vi "Pagina gestione password.vi"() -> (0 "pagina out":i16=255)   [LabVIEW 2022 SP3]
uses:
  Labview/Globali.vi
  <vilib>/Utility/file.llb/Read From Spreadsheet File (string).vi
  <vilib>/Utility/file.llb/Write To Spreadsheet File (string).vi
panel:
  in  "Informazioni operatore 2":T1
  out "Manutenzione":string
  out "Autocontrollo Man.":string
  out "Password Man.":string
  out "Password Amm.":string
  out "Autocontrollo Amm.":string
  out "Amministratore":string
  in  "Informazioni operatore":T1
  in  "Aggiungi":bool
  in  "Informazioni operatori":T2(array[cluster])
  in  "stop":bool
  out "Password":string
  out "Autocontrollo":string
  out "Operatore":string
  out "Tipo pagina":string
  out "Indicazioni":string
  out "Picture":picture
  out "Versione SW":dbl=1.0 format="%.2f"
  out "Linea":string="CENTAURO"
  out "Testo allarmi":string caption="ALLARMI"
  out "Testo fase collaudo":string caption="FASE COLLAUDO"
  out "Testo segnalazioni":string caption="SEGNALAZIONI"
  out "Testo messaggi":string caption="MESSAGGI"
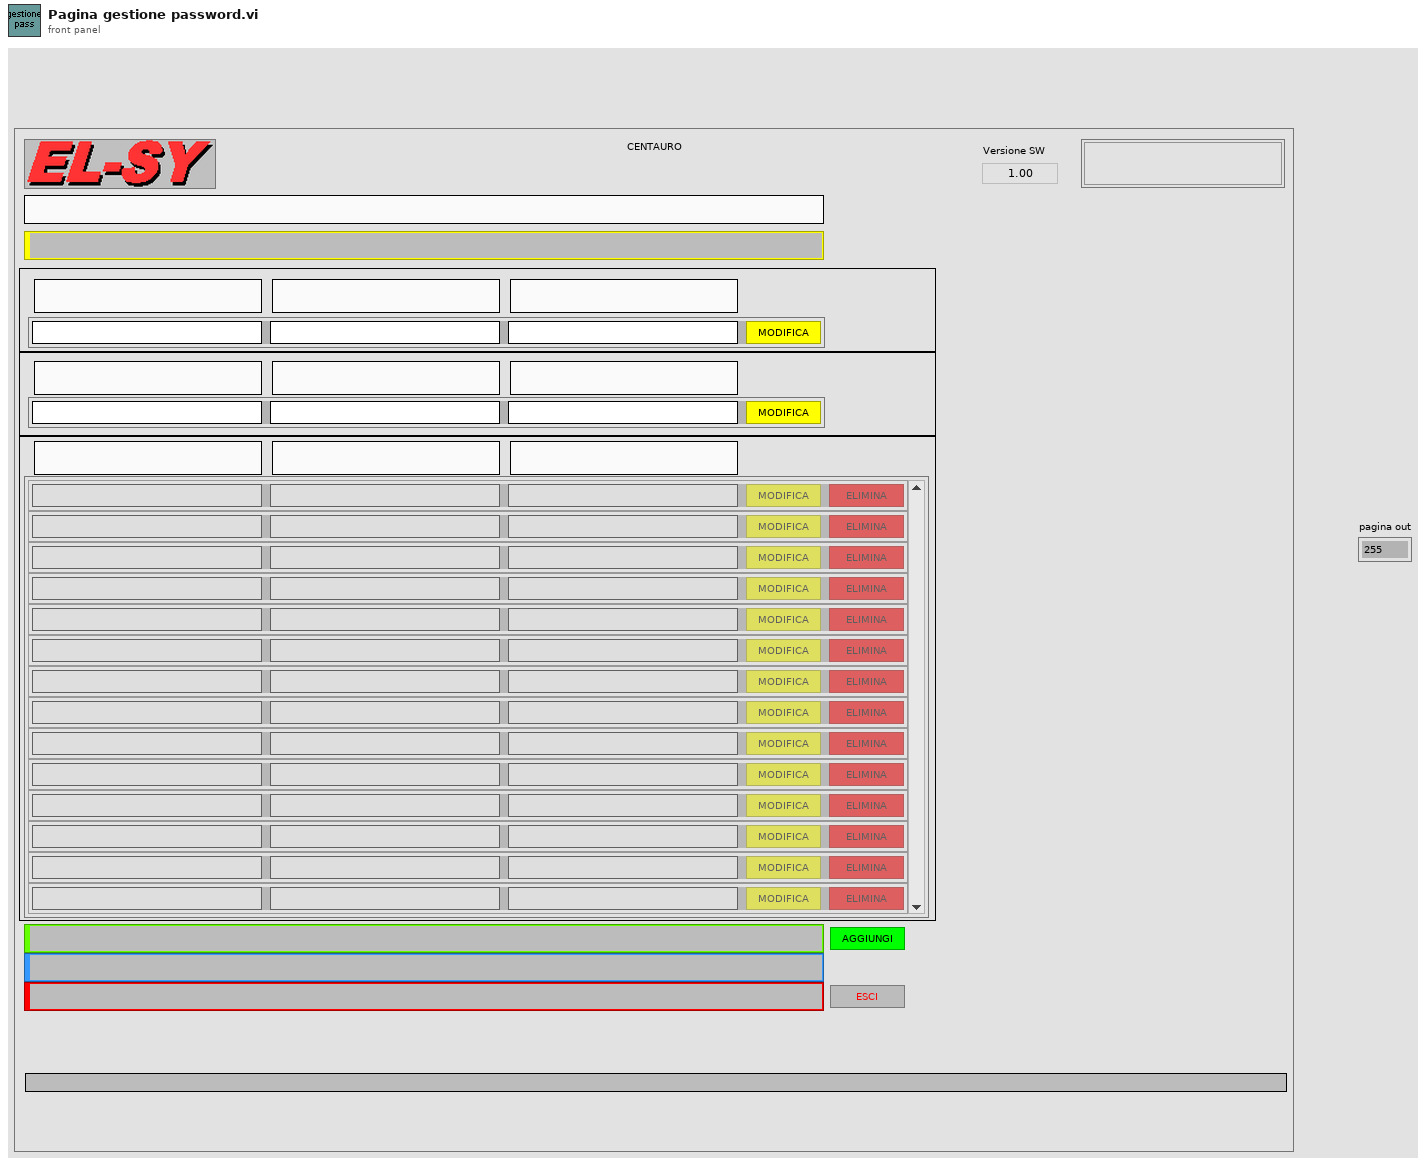
[diagram p1: front panel]
types:
  T1 = cluster{"Operatore":string, "Autocontrollo":string, "Password":string, "Aggiungi":bool, "Modifica":bool, "Elimina":bool}
  T2 = cluster{"Operatore":string, "Autocontrollo":string, "Password":string, "Aggiungi":bool, "Modifica":bool, "Elimina":bool}[]
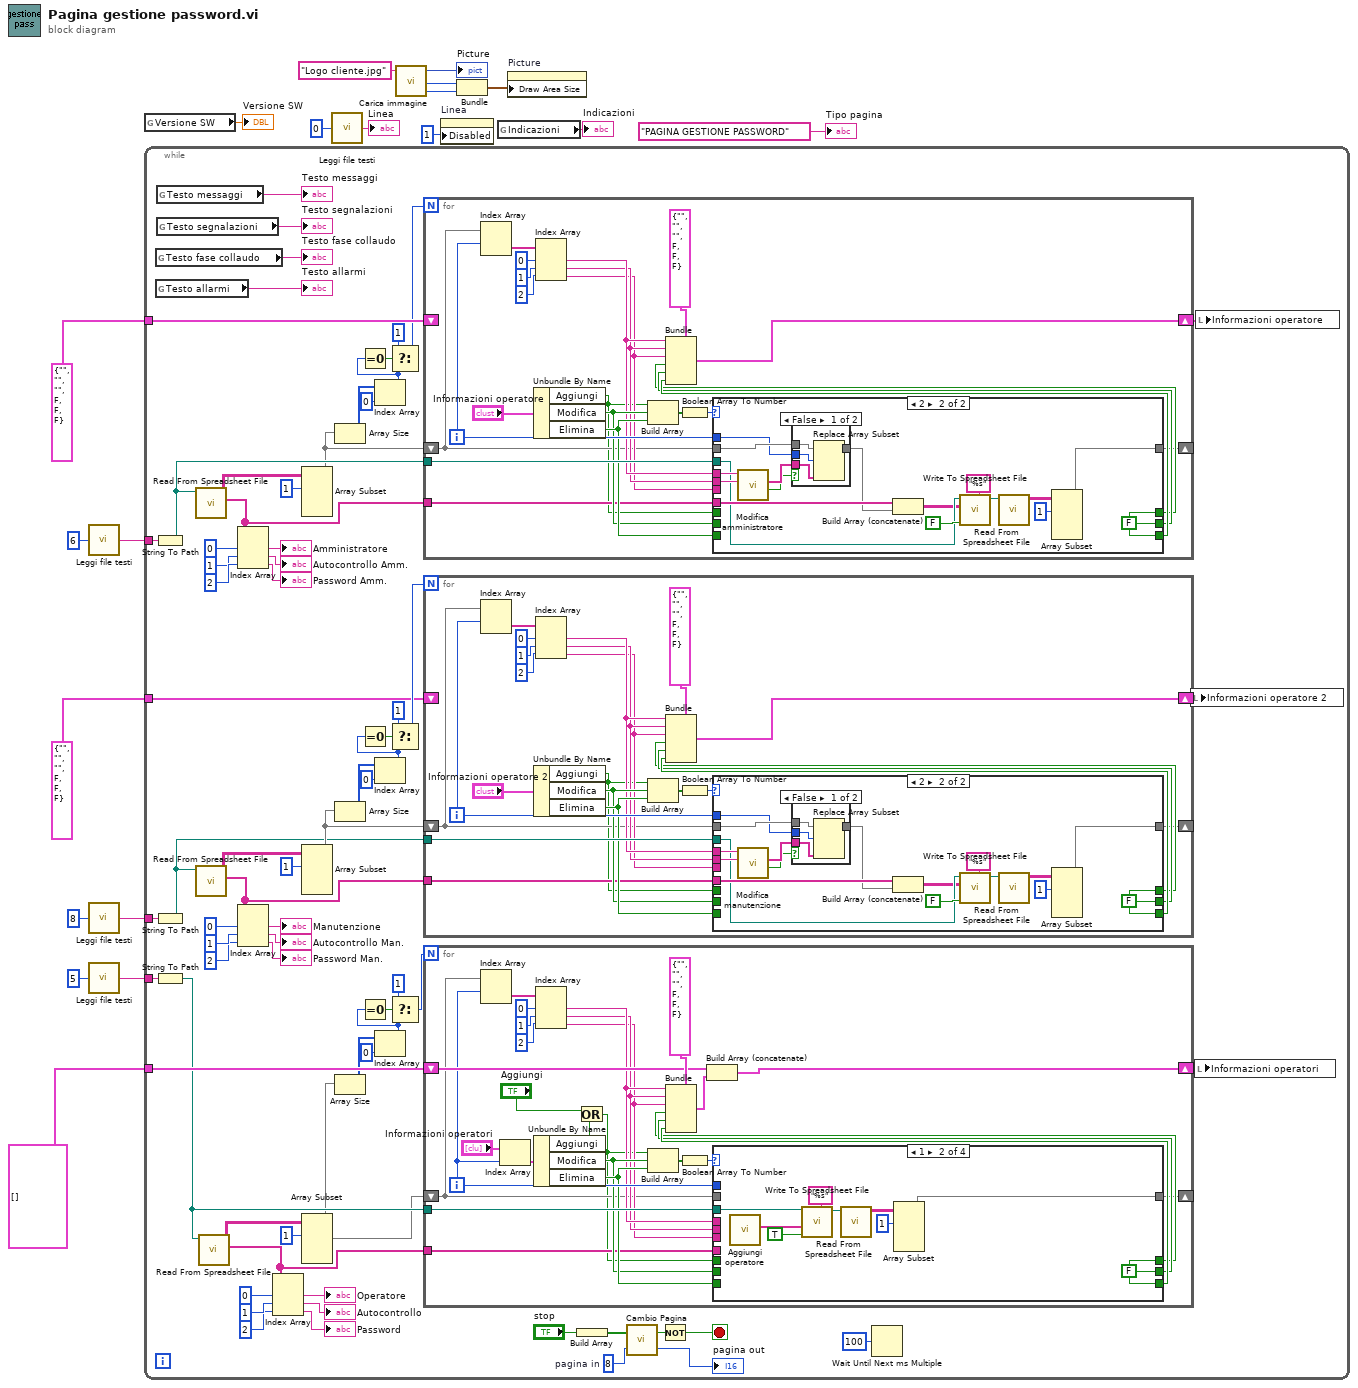
[diagram p0: block diagram]
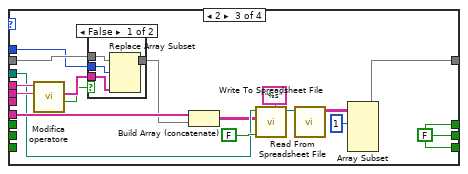
[diagram p7: hidden frame]
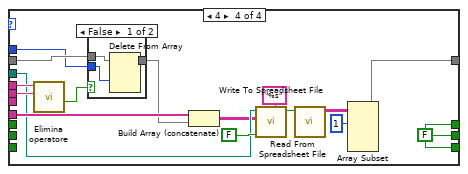
[diagram p9: hidden frame]
diagram:
  n1 = call "Leggi file testi.vi"("Numero riga"=6) -> ("Testo"=w7:string)  [unwired: 3 in, 1 out]
  n2 = call "Leggi file testi.vi"("Numero riga"=8) -> ("Testo"=w1:string)  [unwired: 3 in, 1 out]
  n3 = call "Leggi file testi.vi"("Numero riga"=5) -> ("Testo"=w8:string)  [unwired: 3 in, 1 out]
  n4 = global read "globali.vi" "Versione SW"() -> (→"Versione SW":dbl)
  n5 = while {
    tunnel: w8 -> [w83]
    tunnel: T2 [] ("Informazioni operatori 2") -> [w82]
    tunnel: w7 -> [w61]
    tunnel: T1 {"Operatore"="", "Autocontrollo"="", "Password"="", "Aggiungi"=FALSE, "Modifica"=FALSE, "Elimina"=FALSE} ("Informazioni operatore") -> [w49]
    tunnel: w1 -> [w21]
    tunnel: T1 {"Operatore"="", "Autocontrollo"="", "Password"="", "Aggiungi"=FALSE, "Modifica"=FALSE, "Elimina"=FALSE} ("Informazioni operatore") -> [w32]
    stop <- w62 stop-if-true
    w88 = u8 8  # pagina in
    n6 = String To Path(string=w61) -> (path=w55:path)
    n7 = String To Path(string=w21) -> (path=w27:path)
    n8 = String To Path(string=w83) -> (path=w72:path)
    n9 = global read "Globali.vi" "Testo fase collaudo"() -> (→"Testo fase collaudo":string)
    n10 = global read "Globali.vi" "Testo allarmi"() -> (→"Testo allarmi":string)
    n11 = global read "Globali.vi" "Testo messaggi"() -> (→"Testo messaggi":string)
    n12 = global read "Globali.vi" "Testo segnalazioni"() -> (→"Testo segnalazioni":string)
    n13 = call-poly <vilib>:"Read From Spreadsheet File.vi"("file path (dialog if empty)"=w55) -> ("first row"=w51:string[], "all rows"=w59:string[][])  [unwired: 6 in, 3 out]
    n14 = call-poly <vilib>:"Read From Spreadsheet File.vi"("file path (dialog if empty)"=w27) -> ("first row"=w31:string[], "all rows"=w23:string[][])  [unwired: 6 in, 3 out]
    n15 = call-poly <vilib>:"Read From Spreadsheet File.vi"("file path (dialog if empty)"=w72) -> ("first row"=w50:string[], "all rows"=w75:string[][])  [unwired: 6 in, 3 out]
    n16 = Index Array(array=w51, index #1=0 ("index"), index #2=1 ("index"), index #3=2 ("index")) -> (element #1=→"Amministratore":string, element #2=→"Autocontrollo Amm.":string, element #3=→"Password Amm.":string)
    n17 = Index Array(array=w31, index #1=0 ("index"), index #2=1 ("index"), index #3=2 ("index")) -> (element #1=→"Manutenzione":string, element #2=→"Autocontrollo Man.":string, element #3=→"Password Man.":string)
    n18 = Index Array(array=w50, index #1=0 ("index"), index #2=1 ("index"), index #3=2 ("index")) -> (element #1=→"Operatore":string, element #2=→"Autocontrollo":string, element #3=→"Password":string)
    n19 = Array Subset(array=w59, index (row)=1 ("index")) -> (w41:string[][])  [unwired: 3 in]
    n20 = Array Subset(array=w23, index (row)=1 ("index")) -> (w40:string[][])  [unwired: 3 in]
    n21 = Array Subset(array=w75, index (row)=1 ("index")) -> (w67:string[][])  [unwired: 3 in]
    n22 = Array Size(array=w41) -> (size(s)=w46:i32[])
    n23 = Array Size(array=w40) -> (size(s)=w35:i32[])
    n24 = Array Size(array=w67) -> (size(s)=w66:i32[])
    n25 = Index Array(array=w46, index=0) -> (element=w47:i32)
    n26 = Equal To 0?(x=w47) -> (x = 0?=w44:bool)
    n27 = Index Array(array=w35, index=0) -> (element=w34:i32)
    n28 = Equal To 0?(x=w34) -> (x = 0?=w37:bool)
    n29 = Index Array(array=w66, index=0) -> (element=w65:i32)
    n30 = Equal To 0?(x=w65) -> (x = 0?=w69:bool)
    n31 = Select(t=1, s=w44, f=w47) -> (s? t:f=w42:i32)
    n32 = Select(t=1, s=w37, f=w34) -> (s? t:f=w39:i32)
    n33 = Select(t=1, s=w69, f=w65) -> (s? t:f=w71:i32)
    n34 = for {
      N: w42 -> [_]
      shift-right: [w141] -> w48
      shift-left: w49 -> [_]
      tunnel: w55 -> [w155]
      tunnel: w51 -> [w144]
      shift-right: [w146] -> _
      shift-left: w41 -> [w145]
      i -> [w156]
      n35 = Index Array(array=w145, index (row)=w156) -> (element=w163:string[])  [unwired: 1 in]
      n36 = Unbundle By Name("Informazioni operatore") -> ("Aggiungi"=w142:bool, "Modifica"=w153:bool, "Elimina"=w154:bool)
      n37 = Index Array(array=w163, index #1=0 ("index"), index #2=1 ("index"), index #3=2 ("index")) -> (element #1=w149:string, element #2=w148:string, element #3=w147:string)
      n38 = Build Array(w142, w153, w154) -> (w158:bool[])
      n39 = Boolean Array To Number(Boolean array=w158) -> (number=w157:u32)
      n40 = case shown="2" w157 {
        tunnel: w156 -> [_ w179]
        tunnel: w145 -> [w164 w181]
        tunnel: w155 -> [_ w170]
        tunnel: w154 -> [w165 _]
        tunnel: [w165 w184] -> w152
        tunnel: w142 -> [w167 _]
        tunnel: [w167 w184] -> w150
        tunnel: [w166 w184] -> w151
        tunnel: w153 -> [w166 _]
        tunnel: w149 -> [_ w183]
        tunnel: w148 -> [_ w182]
        tunnel: w147 -> [_ _]
        tunnel: [w164 w168] -> w146
        tunnel: w144 -> [_ w177]
        frame 0, Default {
        }
        frame 2 {
          w184 = FALSE ("Modifica")
          n41 = call "Modifica amministratore.vi"("Autocontrollo"=w182, "Amministratore"=w183) -> ("Annulla?"=w178:bool, "Info amm."=w180:string[])  [unwired: 8 in]
          n42 = case shown="False" w178 {
            tunnel: w181 -> [w188 w189]
            tunnel: w180 -> [w187 _]
            tunnel: w179 -> [w186 _]
            tunnel: [w185 w189] -> w176
            frame False {
              n43 = Replace Array Subset(array=w188, new element=w187, index (row)=w186) -> (w185:string[][])  [unwired: 1 in]
            }
            frame True {
            }
          }
          n44 = Build Array (concatenate)(w177, w176) -> (w169:string[][])
          n45 = call-poly <vilib>:"Write To Spreadsheet File.vi"("format (%s)"="%s" ("format (%.3f)"), "append to file? (new file:F)"=FALSE, "2D data"=w169, "file path (dialog if empty)"=w170) -> ("new file path (Not A Path if cancelled)"=w173:path)  [unwired: 4 in]
          n46 = call-poly <vilib>:"Read From Spreadsheet File.vi"("file path (dialog if empty)"=w173) -> ("all rows"=w171:string[][])  [unwired: 6 in, 4 out]
          n47 = Array Subset(array=w171, index (row)=1 ("index")) -> (w168:string[][])  [unwired: 3 in]
        }
      }
      n48 = Bundle(cluster=T1 {"Operatore"="", "Autocontrollo"="", "Password"="", "Aggiungi"=FALSE, "Modifica"=FALSE, "Elimina"=FALSE} ("Informazioni operatore"), "Operatore"=w149, "Autocontrollo"=w148, "Password"=w147, "Aggiungi"=w150, "Modifica"=w151, "Elimina"=w152) -> (w141:T1)
    }
    n49 = for {
      N: w39 -> [_]
      shift-right: [w92] -> w33
      shift-left: w32 -> [_]
      tunnel: w27 -> [w106]
      tunnel: w31 -> [w95]
      shift-right: [w97] -> _
      shift-left: w40 -> [w96]
      i -> [w107]
      n50 = Index Array(array=w96, index (row)=w107) -> (element=w114:string[])  [unwired: 1 in]
      n51 = Unbundle By Name("Informazioni operatore 2") -> ("Aggiungi"=w93:bool, "Modifica"=w104:bool, "Elimina"=w105:bool)
      n52 = Index Array(array=w114, index #1=0 ("index"), index #2=1 ("index"), index #3=2 ("index")) -> (element #1=w100:string, element #2=w99:string, element #3=w98:string)
      n53 = Build Array(w93, w104, w105) -> (w109:bool[])
      n54 = Boolean Array To Number(Boolean array=w109) -> (number=w108:u32)
      n55 = case shown="2" w108 {
        tunnel: w107 -> [_ w130]
        tunnel: w96 -> [w115 w132]
        tunnel: w106 -> [_ w121]
        tunnel: w105 -> [w116 _]
        tunnel: [w116 w135] -> w103
        tunnel: w93 -> [w118 _]
        tunnel: [w118 w135] -> w101
        tunnel: [w117 w135] -> w102
        tunnel: w104 -> [w117 _]
        tunnel: w100 -> [_ w134]
        tunnel: w99 -> [_ w133]
        tunnel: w98 -> [_ _]
        tunnel: [w115 w119] -> w97
        tunnel: w95 -> [_ w128]
        frame 0, Default {
        }
        frame 2 {
          w135 = FALSE ("Modifica")
          n56 = call "Modifica manutenzione.vi"("Autocontrollo"=w133, "Amministratore"=w134) -> ("Annulla?"=w129:bool, "Info amm."=w131:string[])  [unwired: 8 in]
          n57 = case shown="False" w129 {
            tunnel: w132 -> [w139 w140]
            tunnel: w131 -> [w138 _]
            tunnel: w130 -> [w137 _]
            tunnel: [w136 w140] -> w127
            frame False {
              n58 = Replace Array Subset(array=w139, new element=w138, index (row)=w137) -> (w136:string[][])  [unwired: 1 in]
            }
            frame True {
            }
          }
          n59 = Build Array (concatenate)(w128, w127) -> (w120:string[][])
          n60 = call-poly <vilib>:"Write To Spreadsheet File.vi"("format (%s)"="%s" ("format (%.3f)"), "append to file? (new file:F)"=FALSE, "2D data"=w120, "file path (dialog if empty)"=w121) -> ("new file path (Not A Path if cancelled)"=w124:path)  [unwired: 4 in]
          n61 = call-poly <vilib>:"Read From Spreadsheet File.vi"("file path (dialog if empty)"=w124) -> ("all rows"=w122:string[][])  [unwired: 6 in, 4 out]
          n62 = Array Subset(array=w122, index (row)=1 ("index")) -> (w119:string[][])  [unwired: 3 in]
        }
      }
      n63 = Bundle(cluster=T1 {"Operatore"="", "Autocontrollo"="", "Password"="", "Aggiungi"=FALSE, "Modifica"=FALSE, "Elimina"=FALSE} ("Informazioni operatore"), "Operatore"=w100, "Autocontrollo"=w99, "Password"=w98, "Aggiungi"=w101, "Modifica"=w102, "Elimina"=w103) -> (w92:T1)
    }
    n64 = for {
      N: w71 -> [_]
      shift-right: [w217] -> w73
      shift-left: w82 -> [w211]
      tunnel: w72 -> [w204]
      tunnel: w50 -> [w193]
      shift-right: [w195] -> _
      shift-left: w67 -> [w194]
      i -> [w205]
      n65 = Index Array(array=w194, index (row)=w205) -> (element=w216:string[])  [unwired: 1 in]
      n66 = Index Array(array="Informazioni operatori", index=w205) -> (element=w209:T1)
      n67 = Unbundle By Name(w209) -> ("Aggiungi"=w192:bool, "Modifica"=w202:bool, "Elimina"=w203:bool)
      n68 = Index Array(array=w216, index #1=0 ("index"), index #2=1 ("index"), index #3=2 ("index")) -> (element #1=w198:string, element #2=w197:string, element #3=w196:string)
      n69 = Or(x="Aggiungi", y=w192) -> (x .or. y?=w191:bool)
      n70 = Build Array(w191, w202, w203) -> (w207:bool[])
      n71 = Boolean Array To Number(Boolean array=w207) -> (number=w206:u32)
      n72 = case shown="1" w206 {
        tunnel: w205 -> [_ _ w242 w264]
        tunnel: w194 -> [w218 _ w244 w265]
        tunnel: w204 -> [_ w229 w233 w255]
        tunnel: w203 -> [w219 _ _ _]
        tunnel: [w219 w227 w247 w268] -> w201
        tunnel: w191 -> [w221 _ _ _]
        tunnel: [w221 w227 w247 w268] -> w199
        tunnel: [w220 w227 w247 w268] -> w200
        tunnel: w202 -> [w220 _ _ _]
        tunnel: w198 -> [_ _ w246 w267]
        tunnel: w197 -> [_ _ w245 w266]
        tunnel: w196 -> [_ _ _ _]
        tunnel: [w218 w222 w231 w253] -> w195
        tunnel: w193 -> [_ _ w240 w262]
        frame 0, Default {
        }
        frame 1 {
          w227 = FALSE ("Modifica")
          n73 = call "Aggiungi operatore.vi"() -> ("Info oper."=w226:string[])  [unwired: 11 in]
          n74 = call-poly <vilib>:"Write To Spreadsheet File.vi"("format (%s)"="%s" ("format (%.3f)"), "append to file? (new file:F)"=TRUE, "1D data"=w226, "file path (dialog if empty)"=w229) -> ("new file path (Not A Path if cancelled)"=w225:path)  [unwired: 4 in]
          n75 = call-poly <vilib>:"Read From Spreadsheet File.vi"("file path (dialog if empty)"=w225) -> ("all rows"=w223:string[][])  [unwired: 6 in, 4 out]
          n76 = Array Subset(array=w223, index (row)=1 ("index")) -> (w222:string[][])  [unwired: 3 in]
        }
        frame 2 {
          w247 = FALSE ("Modifica")
          n77 = call "Modifica operatore.vi"("Autocontrollo"=w245, "Operatore"=w246) -> ("Annulla?"=w241:bool, "Info oper."=w243:string[])  [unwired: 8 in]
          n78 = case shown="False" w241 {
            tunnel: w244 -> [w251 w252]
            tunnel: w243 -> [w250 _]
            tunnel: w242 -> [w249 _]
            tunnel: [w248 w252] -> w239
            frame False {
              n79 = Replace Array Subset(array=w251, new element=w250, index (row)=w249) -> (w248:string[][])  [unwired: 1 in]
            }
            frame True {
            }
          }
          n80 = Build Array (concatenate)(w240, w239) -> (w232:string[][])
          n81 = call-poly <vilib>:"Write To Spreadsheet File.vi"("format (%s)"="%s" ("format (%.3f)"), "append to file? (new file:F)"=FALSE, "2D data"=w232, "file path (dialog if empty)"=w233) -> ("new file path (Not A Path if cancelled)"=w236:path)  [unwired: 4 in]
          n82 = call-poly <vilib>:"Read From Spreadsheet File.vi"("file path (dialog if empty)"=w236) -> ("all rows"=w234:string[][])  [unwired: 6 in, 4 out]
          n83 = Array Subset(array=w234, index (row)=1 ("index")) -> (w231:string[][])  [unwired: 3 in]
        }
        frame 4 {
          w268 = FALSE ("Modifica")
          n84 = call "Elimina operatore.vi"("Autocontrollo"=w266, "Operatore"=w267) -> ("Annulla?"=w263:bool)  [unwired: 8 in, 1 out]
          n85 = case shown="False" w263 {
            tunnel: w265 -> [w271 w272]
            tunnel: w264 -> [w269 _]
            tunnel: [w270 w272] -> w261
            frame False {
              n86 = Delete From Array(array=w271, index (row)=w269) -> (array with subset deleted=w270:string[][])  [unwired: 2 in, 1 out]
            }
            frame True {
            }
          }
          n87 = Build Array (concatenate)(w262, w261) -> (w254:string[][])
          n88 = call-poly <vilib>:"Write To Spreadsheet File.vi"("format (%s)"="%s" ("format (%.3f)"), "append to file? (new file:F)"=FALSE, "2D data"=w254, "file path (dialog if empty)"=w255) -> ("new file path (Not A Path if cancelled)"=w258:path)  [unwired: 4 in]
          n89 = call-poly <vilib>:"Read From Spreadsheet File.vi"("file path (dialog if empty)"=w258) -> ("all rows"=w256:string[][])  [unwired: 6 in, 4 out]
          n90 = Array Subset(array=w256, index (row)=1 ("index")) -> (w253:string[][])  [unwired: 3 in]
        }
      }
      n91 = Bundle(cluster=T1 {"Operatore"="", "Autocontrollo"="", "Password"="", "Aggiungi"=FALSE, "Modifica"=FALSE, "Elimina"=FALSE} ("Informazioni operatore"), "Operatore"=w198, "Autocontrollo"=w197, "Password"=w196, "Aggiungi"=w199, "Modifica"=w200, "Elimina"=w201) -> (w210:T1)
      n92 = Build Array (concatenate)(w211, w210) -> (w217:T2)
    }
    n93 = Build Array("stop") -> (w64:bool[])
    n94 = call "Cambio Pagina.vi"("pagina in"=w88, "pulsanti"=w64) -> ("pagina out"=→"pagina out":u8, "premuto"=w90:bool)
    n95 = Not(x=w90) -> (.not. x?=w62:bool)
    n96 = Wait Until Next ms Multiple(millisecond multiple=u32 100) -> ()  [unwired: 1 out]
    n97 = local write "Informazioni operatore 2"(w33) -> ()
    n98 = local write "Informazioni operatori"(w73) -> ()
    n99 = local write "Informazioni operatore"(w48) -> ()
  }
  n100 = call "Leggi file testi.vi"("Numero riga"=0) -> ("Testo"=→"Linea":string)  [unwired: 3 in, 1 out]
  n101 = call "Carica immagine.vi"("Immagine JPG"="Logo cliente.jpg") -> ("altezza"=w16:i16, "larghezza"=w17:i16, "Picture"=→"Picture":picture)  [unwired: 2 in]
  n102 = property on="Linea" class="Str"("Disabled"=u8 1) -> ()  [unwired: 2 in, 2 out]
  n103 = Bundle("larghezza"=w17, "altezza"=w16) -> (w15:cluster{"larghezza":i16, "altezza":i16})  [unwired: 1 in]
  n104 = global read "Globali.vi" "Indicazioni"() -> (→"Indicazioni":string)
  n105 = property on="Picture" class="Pict"("Draw Area Size"=w15) -> ()  [unwired: 2 in, 2 out]
  "Tipo pagina" <- "PAGINA GESTIONE PASSWORD" ("Tipo pagina")
